vi "PWM, DIO.vi"(6 "Enum":enum16{"M4", "M3", "M2", "M1"}(ring), 8 "error in (no error)":errorcluster, 9 "PWM":dbl) -> (0 "error out 2":errorcluster)   [LabVIEW 2018]
uses:
  <vilib>/Utility/error.llb/Error Cluster From Error Code.vi
  <vilib>/myRIO/Common/Instrument Driver Framework/myRIO v1.0/PWM/vis/myRIO v1.0 Write PWM.vi
  <vilib>/myRIO/Common/Instrument Driver Framework/myRIO v1.0/DIO/vis/myRIO v1.0 Write DIO.vi
  <vilib>/myRIO/Instrument Drivers/Onboard IO/PWM/PWM.lvlib
  <vilib>/myRIO/Instrument Drivers/Onboard IO/DIO/DIO.lvlib
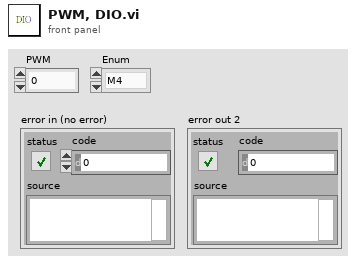
[diagram p1: front panel]
types:
  T1 = typedef "PWM.lvlib/PWM Reference.ctl" = cluster{"myRIO Reference":T2, "PWM Channels Enum":T6, "PWM Configuration":T7}
  T2 = typedef "myRIO Generic Hardware Reference.ctl" = cluster{"myRIO Model":T3, "myRIO Hardware Reference":T4}
  T3 = typedef "Hardware Version Enum.ctl" = enum16{"Unknown", "myRIO-1900", "myRIO-1950", "roboRIO", "NI ELVIS RIO CM", "ELVIS III"}
  T4 = typedef "myRIO v1.0 Reference.ctl" = cluster{"Generic FPGA Reference":T5, "Allow multiple opens":bool}
  T5 = typedef "Generic FPGA Reference.ctl" = refnum<k20>
  T6 = typedef "PWM Channels Enum.ctl" = enum16{"Not Connected", "C/PWM0", "C/PWM1", "A/PWM0", "A/PWM1", "A/PWM2", "A/PWM3", "A/PWM4", "A/PWM5", "A/PWM6", "A/PWM7", "A/PWM8", "A/PWM9", "A/PWM10", "A/PWM11", "A/PWM12", "A/PWM13", "A/PWM14", "A/PWM15", "A/PWM16", "A/PWM17", "A/PWM18", "A/PWM19", "B/PWM0", "B/PWM1", "B/PWM2", "B/PWM3", "B/PWM4", "B/PWM5", "B/PWM6", "B/PWM7", "B/PWM8", "B/PWM9", "B/PWM10", "B/PWM11", "B/PWM12", "B/PWM13", "B/PWM14", "B/PWM15", "B/PWM16", "B/PWM17", "B/PWM18", "B/PWM19", "PWM/PWM0", "PWM/PWM1", "PWM/PWM2", "PWM/PWM3", "PWM/PWM4", "PWM/PWM5", "PWM/PWM6", "PWM/PWM7", "PWM/PWM8", "PWM/PWM9"}
  T7 = typedef "PWM.lvlib/PWM Configuration.ctl" = cluster{"Frequency":dbl, "Duty Cycle":dbl}
  T8 = typedef "DIO.lvlib/DIO Reference.ctl" = cluster{"myRIO Reference":T2, "DIO Channels List":T9}
  T9 = typedef "DIO Channels List.ctl" = T10[]
  T10 = typedef "DIO Channels Enum.ctl" = enum16{"Not Connected", "C/DIO0", "C/DIO1", "C/DIO2", "C/DIO3", "C/DIO4", "C/DIO5", "C/DIO6", "C/DIO7", "A/DIO0", "A/DIO1", "A/DIO2", "A/DIO3", "A/DIO4", "A/DIO5", "A/DIO6", "A/DIO7", "A/DIO8", "A/DIO9", "A/DIO10", "A/DIO11", "A/DIO12", "A/DIO13", "A/DIO14", "A/DIO15", "A/DIO16", "A/DIO17", "A/DIO18", "A/DIO19", "B/DIO0", "B/DIO1", "B/DIO2", "B/DIO3", "B/DIO4", "B/DIO5", "B/DIO6", "B/DIO7", "B/DIO8", "B/DIO9", "B/DIO10", "B/DIO11", "B/DIO12", "B/DIO13", "B/DIO14", "B/DIO15", "B/DIO16", "B/DIO17", "B/DIO18", "B/DIO19", "LED0", "LED1", "LED2", "LED3", "Button0", "DIO/DIO0", "DIO/DIO1", "DIO/DIO2", "DIO/DIO3", "DIO/DIO4", "DIO/DIO5", "DIO/DIO6", "DIO/DIO7", "DIO/DIO8", "DIO/DIO9", "SPI/CS0", "SPI/CS1", "SPI/CS2", "SPI/CS3", "LED RADIO (Green)", "LED RADIO (Red)", "LED COMM (Green)", "LED COMM (Red)", "LED MODE (Green)", "LED MODE (Red)"}
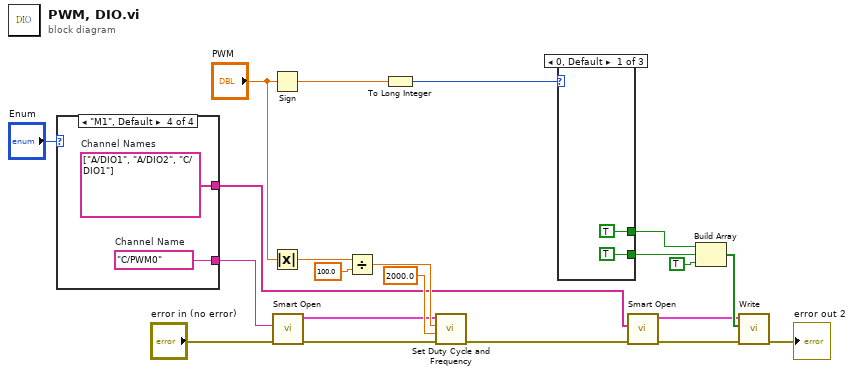
[diagram p0: block diagram]
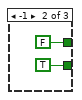
[diagram p2: hidden frame]
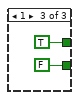
[diagram p3: hidden frame]
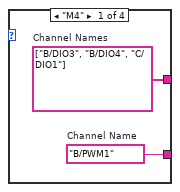
[diagram p4: hidden frame]
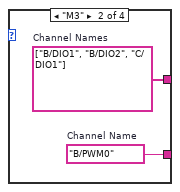
[diagram p5: hidden frame]
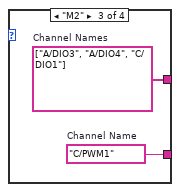
[diagram p6: hidden frame]
diagram:
  n1 = case shown="\"M1\", Default" "Enum" {
    tunnel: [w23 w25 w27 w29] -> w13
    tunnel: [w22 w24 w26 w28] -> w5
    frame "M4" {
      w22 = tag[] ["B/DIO3", "B/DIO4", "C/DIO1"]  # Channel Names
      w23 = tag "B/PWM1"  # Channel Name
    }
    frame "M3" {
      w24 = tag[] ["B/DIO1", "B/DIO2", "C/DIO1"]  # Channel Names
      w25 = tag "B/PWM0"  # Channel Name
    }
    frame "M2" {
      w26 = tag[] ["A/DIO3", "A/DIO4", "C/DIO1"]  # Channel Names
      w27 = tag "C/PWM1"  # Channel Name
    }
    frame "M1", Default {
      w28 = tag[] ["A/DIO1", "A/DIO2", "C/DIO1"]  # Channel Names
      w29 = tag "C/PWM0"  # Channel Name
    }
  }
  n2 = Sign(1:"PWM") -> (0:w2:dbl)
  n3 = Absolute Value(x="PWM") -> (abs(x)=w14:dbl)
  n4 = call <vilib>:"Smart Open.vi"("error in (no error)"="error in (no error)", "Channel Name"=w13) -> ("error out"=w11:errorcluster, "PWM Ref Out"=w10:T1)  [unwired: 8 in]
  n5 = Divide(x=w14, y=100.0) -> (x/y=w16:dbl)
  n6 = To Long Integer(number=w2) -> (32bit integer=w1:i32)
  n7 = call <vilib>:"Set Duty Cycle and Frequency.vi"("error in (no error)"=w11, "Frequency [Hz]"=2000.0, "Duty Cycle"=w16, "PWM Ref In"=w10) -> ("error out"=w6:errorcluster)  [unwired: 5 in, 1 out]
  n8 = case shown="0, Default" w1 {
    tunnel: [TRUE FALSE ("element") TRUE ("element")] -> w20
    tunnel: [TRUE TRUE ("element") FALSE ("element")] -> w21
    frame 0, Default {
    }
    frame -1 {
    }
    frame 1 {
    }
  }
  n9 = call <vilib>:"Smart Open.vi"("error in (no error)"=w6, "Channel Names"=w5) -> ("error out"=w4:errorcluster, "DIO Ref Out"=w3:T8)  [unwired: 8 in]
  n10 = Build Array(w20, w21, TRUE ("element")) -> (w18:bool[])
  n11 = call <vilib>:"Write.vi"("error in (no error)"=w4, "Values"=w18, "DIO Ref In"=w3) -> ("error out"=→"error out 2":errorcluster)  [unwired: 6 in, 1 out]
